vi "geve-msg_append_to_log.vi"(7 "Priority":bool, 8 "error in (no error)":errorcluster, 10 "Status Message":string, 11 "Runtime Data":T1) -> (0 "error out":errorcluster, 3 "Runtime Dataout":T1)   [LabVIEW 2018]
doc: "send message to append new message to log"
uses:
  geve-runtime_data_cluster.ctl
  geve-monitoring_data_cluster.ctl
  geve-serial_config_cluster.ctl
  geve-com_ref_cluster.ctl
  geve-message_cluster.ctl
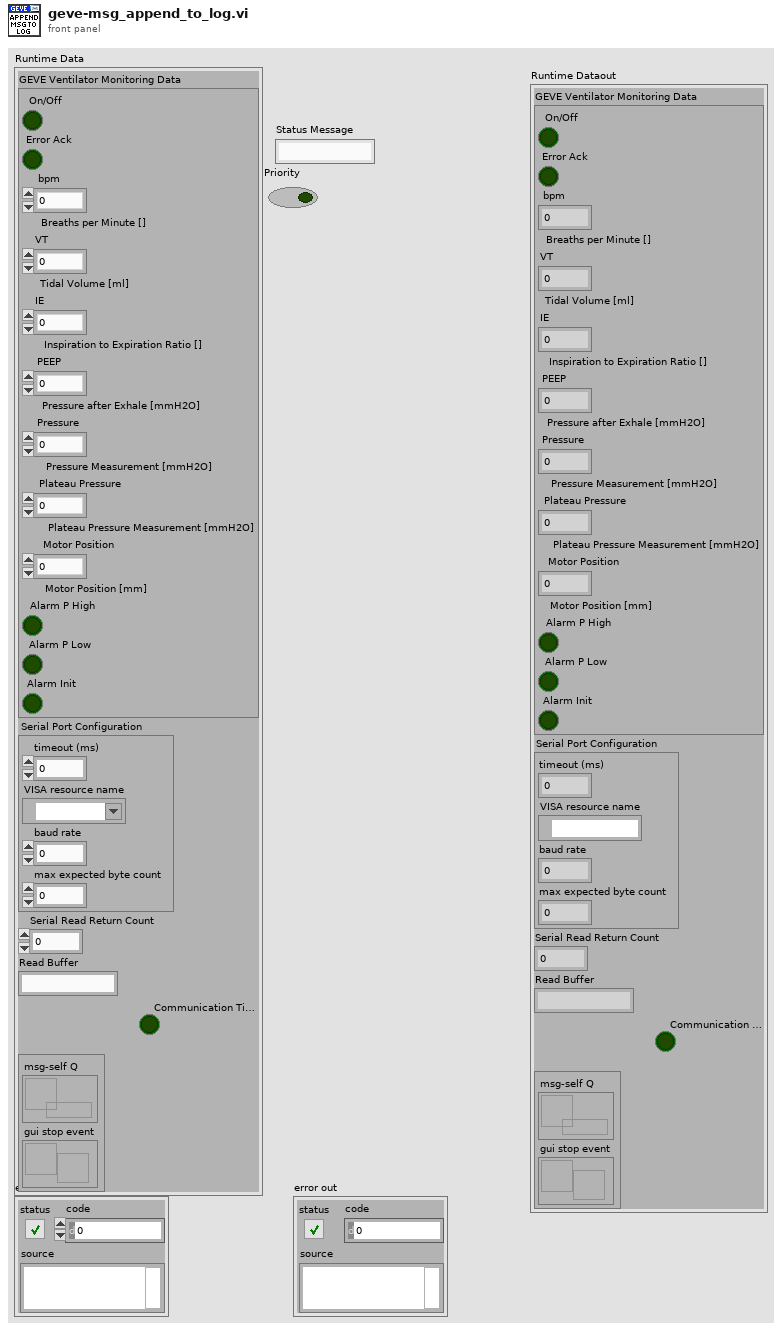
[diagram p1: front panel]
types:
  T1 = typedef "geve-runtime_data_cluster.ctl" = cluster{"GEVE Ventilator Monitoring Data":T2, "Serial Port Configuration":T3, "Serial Read Return Count":u32, "Read Buffer":string, "Communication Timeout?":bool, "com-refs":T4}
  T2 = typedef "geve-monitoring_data_cluster.ctl" = cluster{"On/Off":bool, "Error Ack":bool, "bpm":dbl, "VT":dbl, "IE":dbl, "PEEP":dbl, "Pressure":dbl, "Plateau Pressure":dbl, "Motor Position":dbl, "Alarm P High":bool, "Alarm P Low":bool, "Alarm Init":bool}
  T3 = typedef "geve-serial_config_cluster.ctl" = cluster{"timeout (ms)":u32, "VISA resource name":refnum<visa-resource-name>, "baud rate":u32, "max expected byte count":u32}
  T4 = typedef "geve-com_ref_cluster.ctl" = cluster{"msg-self Q":refnum<queue>, "gui stop event":refnum<user-event>}
  T5 = typedef "geve-message_cluster.ctl" = cluster{"Command":string, "Payload":variant}
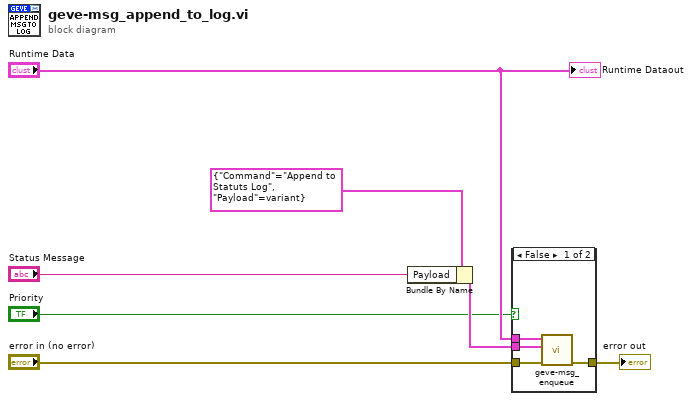
[diagram p0: block diagram]
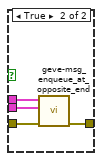
[diagram p2: hidden frame]
diagram:
  n1 = Bundle By Name(cluster=T5 {"Command"="Append to Statuts Log", "Payload"=variant} ("Message"), "Payload"="Status Message") -> (w3:T5)
  n2 = case shown="False" "Priority" {
    tunnel: [w11 w15] -> w7
    tunnel: "error in (no error)" -> [w10 w14]
    tunnel: "Runtime Data" -> [w9 w13]
    tunnel: w3 -> [w8 w12]
    frame False {
      n3 = call "geve-msg_enqueue.vi"("error in (no error)"=w10, "Message"=w8, "Runtime Data"=w9) -> ("error out"=w11:errorcluster)  [unwired: 7 in, 1 out]
    }
    frame True {
      n4 = call "geve-msg_enqueue_at_opposite_end.vi"("error in (no error)"=w14, "Message"=w12, "Runtime Data"=w13) -> ("error out"=w15:errorcluster)  [unwired: 8 in]
    }
  }
  "error out" <- w7
  "Runtime Dataout" <- "Runtime Data"
